vi "run.vi"(11 "call function by reference in":refnum<class "call function by reference.lvclass">) -> (2 "result":refnum<class "result.lvclass">, 3 "call function by reference out":refnum<class "call function by reference.lvclass">)   [LabVIEW 2013, in "call function by reference.lvclass"]
uses:
  call function by reference.lvclass
  result/result.lvclass
  call function by reference.lvclass/call function by reference.ctl
  task/task.lvclass/task.ctl
  task/task.lvclass
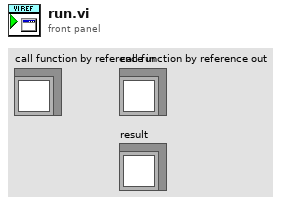
[diagram p1: front panel]
types:
  T1 = typedef "call function by reference.lvclass/function definition.ctl" = refnum<vi>
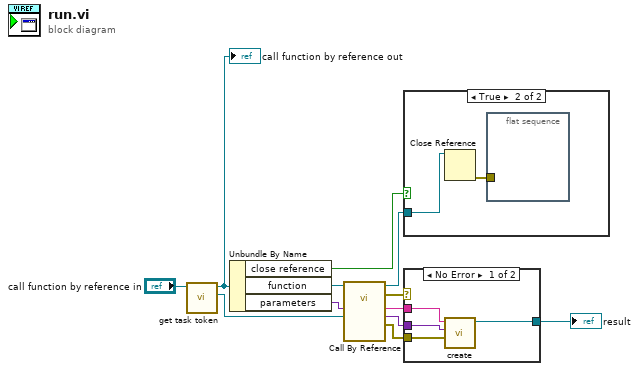
[diagram p0: block diagram]
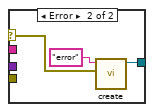
[diagram p3: hidden frame]
diagram:
  n1 = call "get task token.vi"("task in"="call function by reference in") -> ("task token"=w1:refnum<class "null task token.lvclass">, "task out"=w2:refnum<class "call function by reference.lvclass">)  [unwired: 9 in]
  "call function by reference out" <- w2
  n2 = Unbundle By Name(w2) -> ("close reference"=w7:bool, "function"=w12:T1, "parameters"=w3:variant)
  n3 = call-by-ref "?"(reference=w12, "task token"=w1, "parameters"=w3) -> (reference out=w6:T1, error out=w11:errorcluster, "error"=w8:errorcluster, "data"=w9:variant, "data ID"=w10:string)  [unwired: 8 in]
  n4 = case shown="True" w7 {
    tunnel: w6 -> [_ w14]
    frame False {
    }
    frame True {
      n5 = Close Reference(reference=w14) -> (error out=w13:errorcluster)  [unwired: 1 in]
      n6 = flat-sequence {
        tunnel: w13 -> [_]
        frame #0 {
        }
      }
    }
  }
  n7 = case shown="No Error" w11 {
    selector: w11 -> [_ w20]
    tunnel: [w18 w19] -> w4
    tunnel: w10 -> [w17 _]
    tunnel: w9 -> [w16 _]
    tunnel: w8 -> [w15 _]
    frame No Error {
      n8 = call "create.vi"("error"=w15, "data"=w16, "data ID"=w17) -> ("result out"=w18:refnum<class "result.lvclass">)  [unwired: 8 in]
    }
    frame Error {
      n9 = call "create.vi"("data"=w20, "data ID"="error") -> ("result out"=w19:refnum<class "result.lvclass">)  [unwired: 9 in]
    }
  }
  "result" <- w4
